vi "test_variance_map_filtered.vi"() -> ()   [LabVIEW 2009]
doc: "Copyright (c) 2010 Stepan A. Baranov (stepan@baranov.su)\nAll rights reserved.\nweb-site: www.OCTLab.org"
uses:
  <vilib>/Analysis/NI_AALBase.lvlib
  OCTLib_64.dll
panel:
  out "min":dbl format="%0.2f"
  out "max":dbl format="%0.2f"
  out "version":string
  out "name":string
  out "error out":errorcluster
  out "cell height":i32
  out "cell width":i32
  out "A-scan size":i32
  out "# of A-scans":i32
  in  "Small/Big":bool
  out "loop #":i32
  out "RSM_STAT time":u32
  out "LabView time":u32
  out "RSM_STAT Array":dbl[][](array[numeric])
  out "LabView Array":dbl[][](array[numeric])
  in  "stop":bool
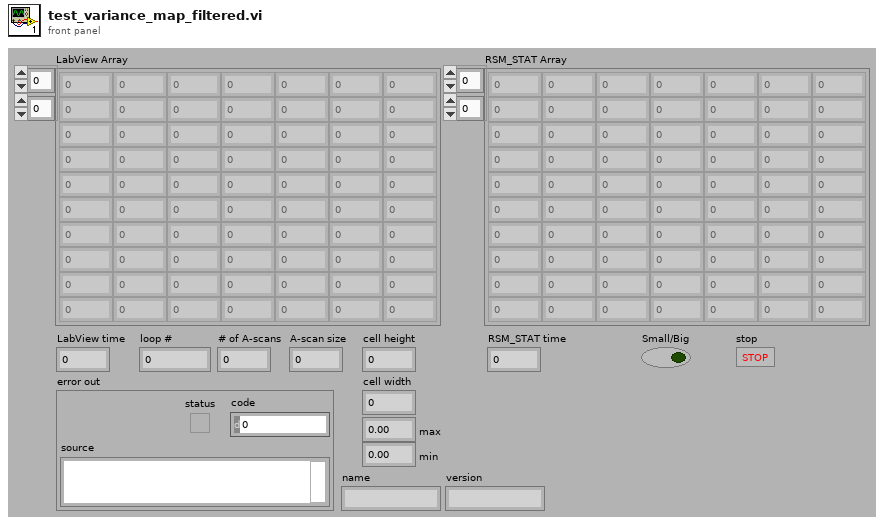
[diagram p1: front panel]
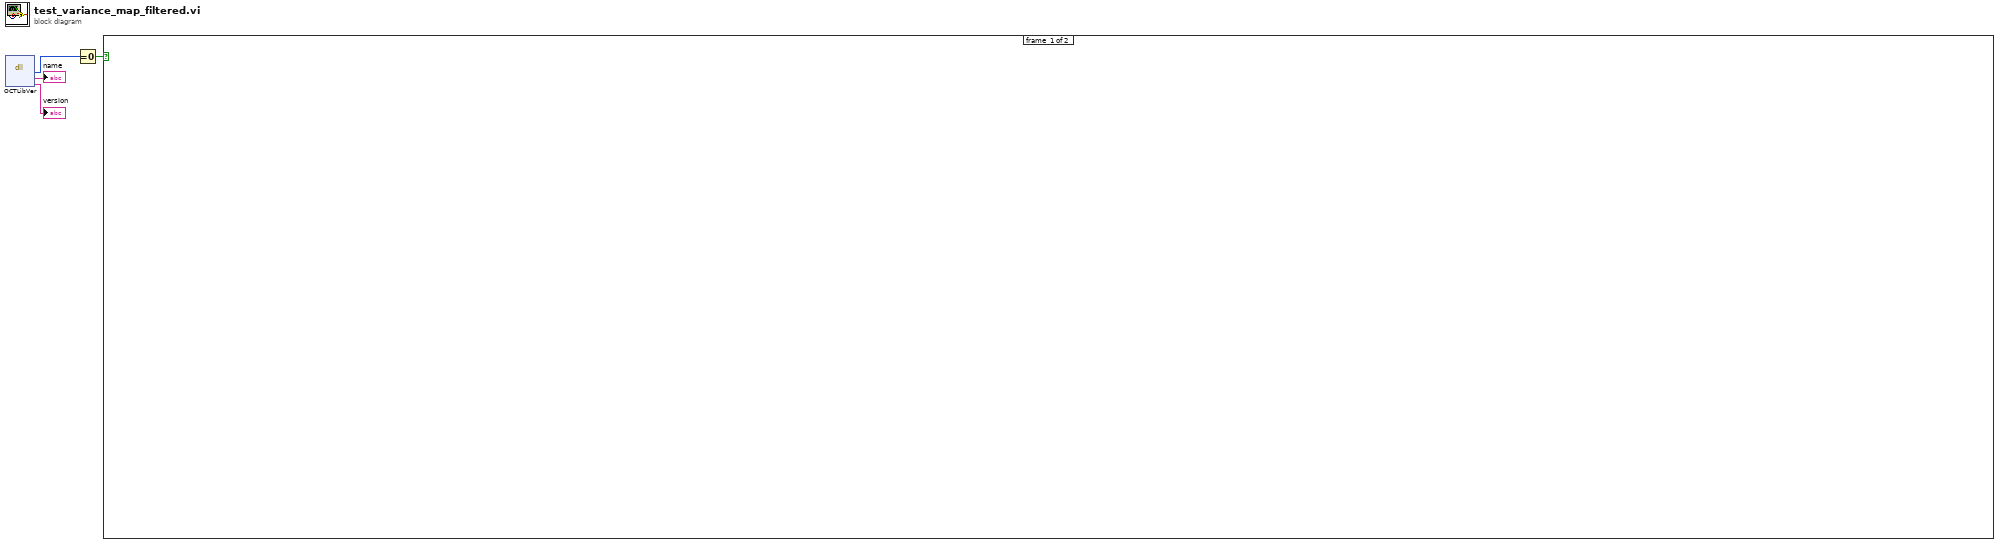
[diagram p0: block diagram]
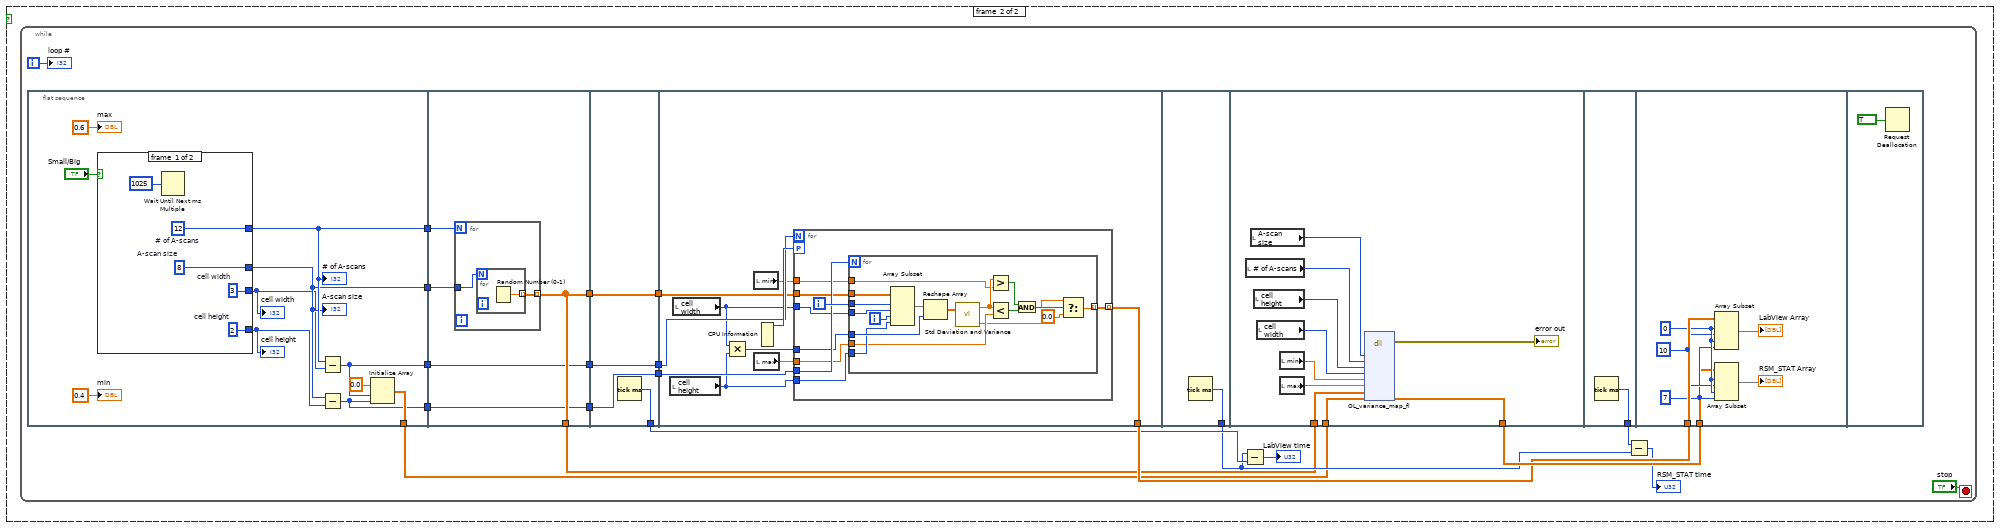
[diagram p2: hidden frame]
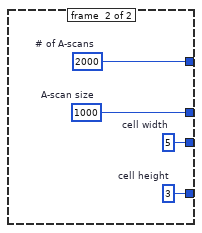
[diagram p3: hidden frame]
diagram:
  n1 = dll-call lib="OCTLib**.*" fn="OCTLibVer"() -> ("status"=w4:i8, "name"=→"name":string, "version"=→"version":string)  [unwired: 5 in, 2 out]
  n2 = Equal To 0?(x=w4) -> (x = 0?=w3:bool)
  n3 = case shown="True" w3 {
    frame #0 {
    }
    frame #1 {
      n4 = while {
        i -> [w17]
        stop <- "stop" stop-if-true
        n5 = flat-sequence {
          tunnel: [w33] -> w13
          tunnel: [w35] -> w12
          tunnel: [w32] -> w11
          tunnel: [w29] -> w6
          tunnel: [w28] -> w5
          tunnel: [w50] -> w16
          tunnel: [w50] -> w14
          tunnel: w13 -> [w49]
          tunnel: w12 -> [w48]
          tunnel: [w46] -> w10
          tunnel: [w47] -> w8
          tunnel: w6 -> [w47]
          tunnel: w5 -> [w46]
          tunnel: [w57] -> w22
          tunnel: [w56] -> w15
          tunnel: w14 -> [w56]
          tunnel: w10 -> [w55]
          tunnel: [w55] -> w9
          tunnel: w8 -> [w54]
          tunnel: [w54] -> w7
          tunnel: [w66] -> w23
          tunnel: w15 -> [w60]
          tunnel: w9 -> [w65]
          tunnel: w7 -> [w64]
          tunnel: [w94] -> w19
          tunnel: w16 -> [w101]
          tunnel: [w104] -> w24
          tunnel: w11 -> [w98]
          tunnel: [w105] -> w20
          tunnel: w24 -> [w106]
          tunnel: w23 -> [w112]
          frame #0 {
            n6 = case shown="False" "Small/Big" {
              tunnel: [w40 w44] -> w35
              tunnel: [w41 w45] -> w33
              tunnel: [w38 w43] -> w30
              tunnel: [w37 w42] -> w31
              frame #0 {
                w37 = 2  # cell height
                w38 = 3  # cell width
                w41 = 8  # A-scan size
                w40 = 12  # # of A-scans
                n7 = Wait Until Next ms Multiple(millisecond multiple=u32 1025) -> ()  [unwired: 1 out]
              }
              frame #1 {
                w42 = 3  # cell height
                w43 = 5  # cell width
                w45 = 1000  # A-scan size
                w44 = 2000  # # of A-scans
              }
            }
            "# of A-scans" <- w35
            "A-scan size" <- w33
            "cell width" <- w30
            "cell height" <- w31
            n8 = Subtract(x=w35, y=w30) -> (x-y=w29:i32)
            n9 = Subtract(x=w33, y=w31) -> (x-y=w28:i32)
            n10 = Initialize Array(0.0 ("element"), w29, w28) -> (w32:dbl[][])
            "max" <- 0.6 ("min")
            "min" <- 0.4 ("min")
          }
          frame #1 {
            n11 = for {
              N: w48 -> [_]
              tunnel: w49 -> [w52]
              tunnel: [w51] -> w50 mode=indexing
              n12 = for {
                N: w52 -> [_]
                tunnel: [w53] -> w51 mode=indexing
                n13 = Random Number (0-1)() -> (number: 0 to 1=w53:dbl)
              }
            }
          }
          frame #2 {
            n14 = Tick Count (ms)() -> (millisecond timer value=w57:u32)
          }
          frame #3 {
            n15 = local read "cell height"() -> (w61:i32)
            n16 = local read "cell width"() -> (w62:i32)
            n17 = Multiply(x=w62, y=w61) -> (x*y=w63:i32)
            n18 = local read "min"() -> (w59:dbl)
            n19 = local read "max"() -> (w58:dbl)
            n20 = CPU Information() -> (4:w67:i32)  [unwired: 3 out]
            n21 = for {
              N: w64 -> [_]
              tunnel: [w75] -> w66 mode=indexing
              workers-P: w67 -> [_]
              tunnel: w65 -> [w74]
              tunnel: w63 -> [w73]
              tunnel: w62 -> [w72]
              tunnel: w61 -> [w71]
              tunnel: w60 -> [w70]
              tunnel: w59 -> [w69]
              tunnel: w58 -> [w68]
              i -> [w76]
              n22 = for {
                N: w74 -> [_]
                tunnel: w76 -> [w93]
                tunnel: [w81] -> w75 mode=indexing
                tunnel: w73 -> [w90]
                tunnel: w72 -> [w89]
                tunnel: w71 -> [w88]
                tunnel: w70 -> [w87]
                tunnel: w69 -> [w79]
                tunnel: w68 -> [w78]
                i -> [w92]
                n23 = Array Subset(array=w87, index (row)=w93, length (row)=w89, index (col)=w92, length (col)=w88) -> (w91:dbl[][])
                n24 = Reshape Array(w91, w90) -> (w86:dbl[])
                n25 = call <vilib>:"Std Deviation and Variance.vi"("X"=w86) -> ("mean"=w80:dbl, "variance"=w77:dbl)  [unwired: 1 in, 1 out]
                n26 = Greater?(x=w80, y=w79) -> (0:w84:bool)
                n27 = Less?(x=w80, y=w78) -> (x < y?=w85:bool)
                n28 = And(x=w84, y=w85) -> (x .and. y?=w83:bool)
                n29 = Select(t=w77, s=w83, f=0.0) -> (s? t:f=w81:dbl)
              }
            }
          }
          frame #4 {
            n30 = Tick Count (ms)() -> (millisecond timer value=w94:u32)
          }
          frame #5 {
            n31 = local read "# of A-scans"() -> (w102:i32)
            n32 = local read "A-scan size"() -> (w103:i32)
            n33 = local read "cell height"() -> (w100:i32)
            n34 = local read "cell width"() -> (w99:i32)
            n35 = local read "min"() -> (w96:dbl)
            n36 = local read "max"() -> (w95:dbl)
            n37 = dll-call lib="OCTLib**.*" fn="OL_variance_map_fl"("A-scan size"=w103, "# of A-scan"=w102, "cell height"=w100, "cell width"=w99, "min"=w96, "max"=w95, "input"=w101, "data"=w98) -> (error out=→"error out":errorcluster, "data"=w104:dbl[][])  [unwired: 11 in, 1 out]
          }
          frame #6 {
            n38 = Tick Count (ms)() -> (millisecond timer value=w105:u32)
          }
          frame #7 {
            w109 = 10 ("length")
            w108 = 7 ("length")
            w110 = 0 ("index")
            n39 = Array Subset(array=w112, index (row)=w110, length (row)=w109, index (col)=w110, length (col)=w108) -> (→"LabView Array":dbl[][])
            n40 = Array Subset(array=w106, index (row)=w110, length (row)=w109, index (col)=w110, length (col)=w108) -> (→"RSM_STAT Array":dbl[][])
          }
          frame #8 {
            n41 = Request Deallocation(TRUE ("flag")) -> ()
          }
        }
        n42 = Subtract(x=w19, y=w22) -> (x-y=→"LabView time":u32)
        n43 = Subtract(x=w20, y=w19) -> (x-y=→"RSM_STAT time":u32)
        "loop #" <- w17
      }
    }
  }
